vi "niWLAN - OPPO - 80211abgnGeneration(ref)_bc.vi"(0 "Rx Measurements Settings":T2 {"DSSS Data Rate (Mbps)" items=["1", "2", "5.5 CCK", "5.5 PBCC", "11 CCK", "11 PBCC", "22", "33"]; "OFDM Data Rate (Mbps)" items=["6", "9", "12", "18", "24", "36", "48", "54"]; "80211n PLCP Frame Format" items=["Mixed Format", "Greenfield Format"]; "Standard" items=["80211A/G/J/P OFDM", "80211B/G DSSS", "80211G DSSSOFDM", "80211N MIMOOFDM", "80211AC MIMOOFDM"]}, 5 "Without ACK ?":bool, 7 "Address String":string="00:90:4C:C5:12:38", 11 "error in":errorcluster) -> (4 "Cluster":T1, 15 "error out":errorcluster)   [LabVIEW 2012]
uses:
  TV/RW/Includes/WLAN - TV - RW - INC - Rx_PER_Wfm_Settings.ctl
  <vilib>/RF Toolkits/WLAN/generation/controls/wlanG version control.ctl
  <vilib>/RF Toolkits/WLAN/generation/niWLANG Create Multiple Channel Waveform (IQ Complex Cluster).vi
  <vilib>/RF Toolkits/WLAN/generation/niWLANG Create Single Channel Waveform (IQ Complex Cluster).vi
  <resource>/objmgr/niWLANGeneration.rc
panel:
  out "32bit integer":i32
  out "1/x":dbl
  in  "Boolean":bool
  in  "Idle Time (With Ack)":dbl
  in  "file path":path
  # "Hardware Configuration"
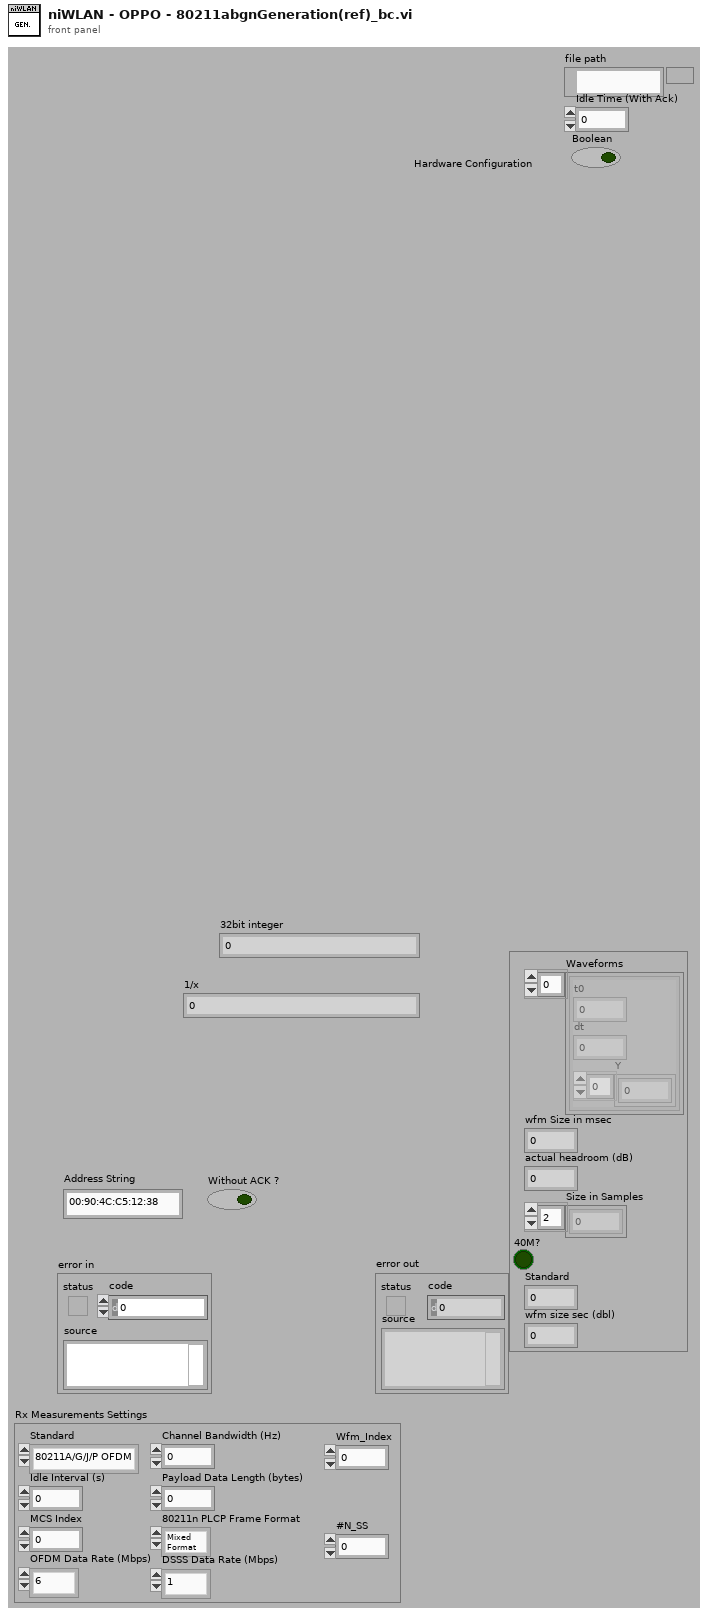
[diagram p1: front panel]
types:
  T1 = cluster{"Waveforms":cluster{"t0":dbl, "dt":dbl, "Y":cdb[]}[], "wfm Size in msec":i32, "actual headroom (dB)":dbl, "Size in Samples":i32[], "40M?":bool, "Standard ":i32, "wfm size sec (dbl)":dbl}
  T2 = typedef "WLAN - TV - RW - INC - Rx_PER_Wfm_Settings.ctl" = cluster{"Standard":i32, "Channel Bandwidth (Hz)":dbl, "Idle Interval (s)":dbl, "MCS Index":i32, "80211n PLCP Frame Format":i32, "Payload Data Length (bytes)":i32, "OFDM Data Rate (Mbps)":i32, "DSSS Data Rate (Mbps)":i32, "Wfm_Index":i32, "#N_SS":i32}
  T3 = typedef "wlanG version control.ctl" = i32
  T4 = typedef "wlanv1_generation refnum.ctl" = refnum<k20>
  T5 = typedef "wlanv1_Generation Refnum.ctl" = refnum<k20>
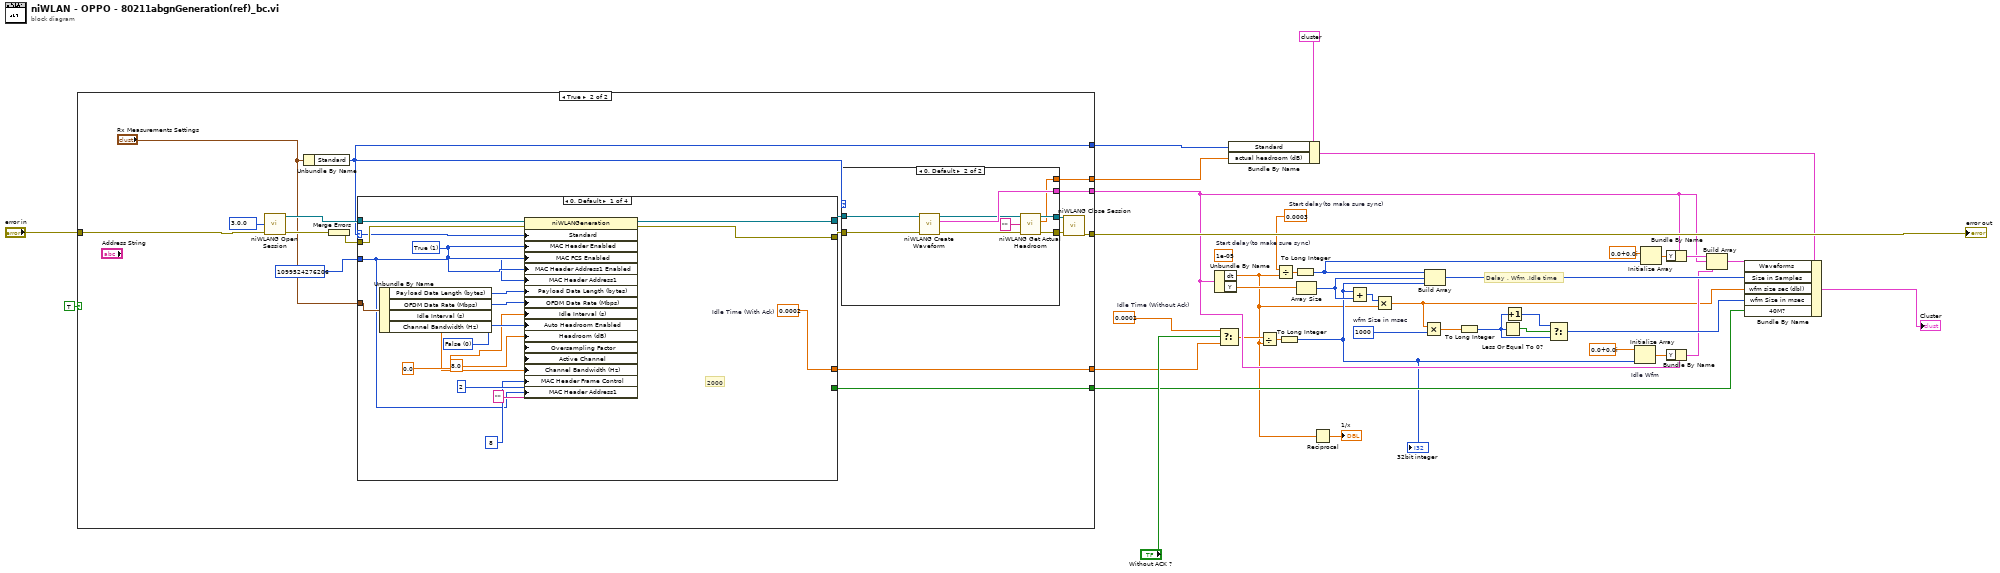
[diagram p0: block diagram]
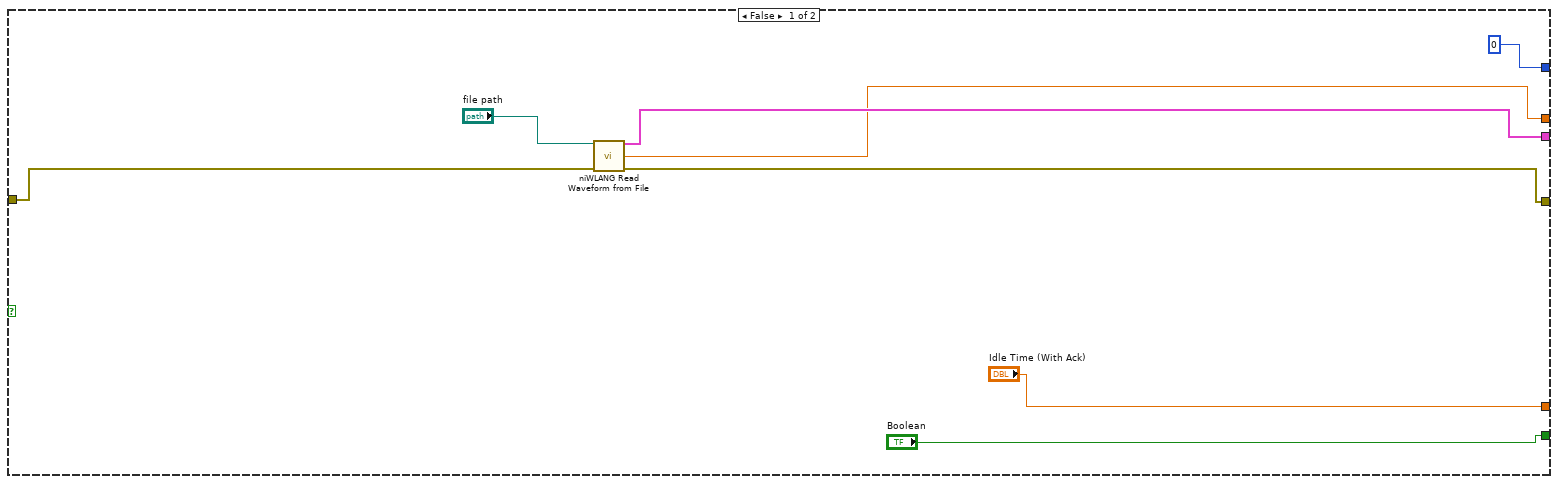
[diagram p2: hidden frame]
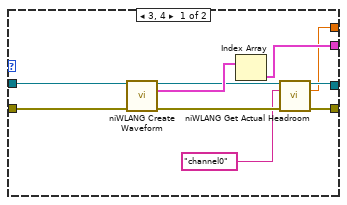
[diagram p3: hidden frame]
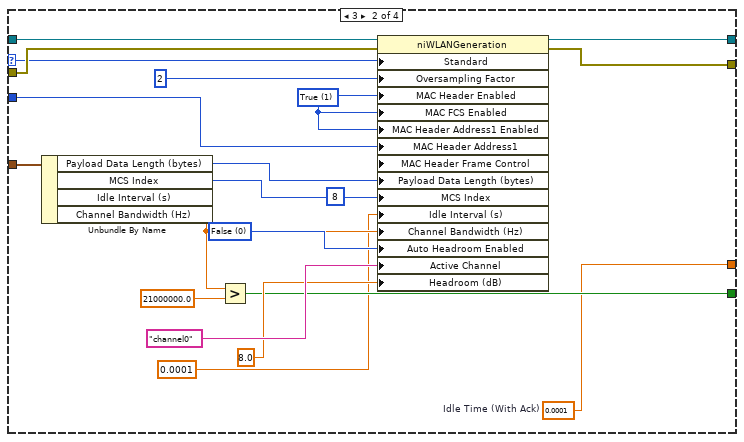
[diagram p4: hidden frame]
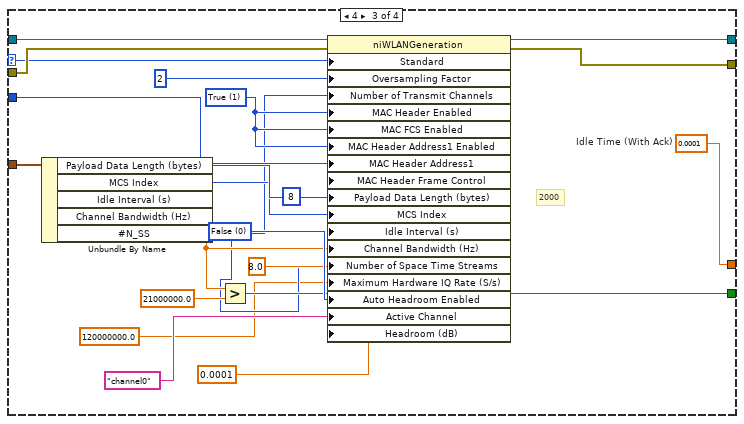
[diagram p5: hidden frame]
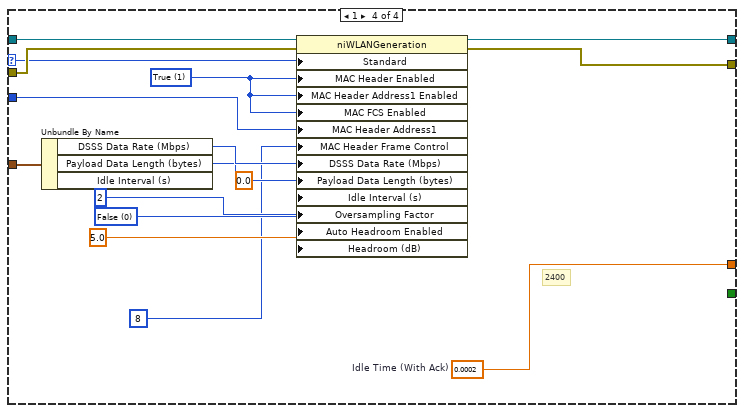
[diagram p6: hidden frame]
diagram:
  w5 = 0.0003  # Start delay(to make sure sync)
  (unwired) 1e-05  # Start delay(to make sure sync)
  w8 = 0.0002  # Idle Time (Without Ack)
  w17 = 1000  # wfm Size in msec
  # "Delay , Wfm ,Idle time"
  n1 = case shown="True" TRUE {
    tunnel: [w44 w64] -> w39
    tunnel: "error in" -> [w41 w63]
    tunnel: ["Boolean" w54] -> w25
    tunnel: [w46 w53] -> w18
    tunnel: [0 ("Standard") w52] -> w12
    tunnel: [w45 w51] -> w10
    tunnel: ["Idle Time (With Ack)" w50] -> w6
    frame False {
      n2 = call <vilib>:"niWLANG Read Waveform from File.vi"("file path"="file path", "error in"=w41) -> ("waveform"=w46:cluster{"t0":dbl, "dt":dbl, "Y":cdb[]}, "headroom (dB)"=w45:dbl, "error out"=w44:errorcluster)  [unwired: 9 in, 2 out]
    }
    frame True {
      w61 = T3 30000 items=["1.0.0"=10000, "2.0.0"=20000, "3.0.0"=30000] ("toolkit compatibility version")
      n3 = call <vilib>:"niWLANG Open Session.vi"("toolkit compatibility version"=w61, "error in"=w63) -> ("niwlan generation session"=w62:T4, "error out"=w60:errorcluster)  [unwired: 11 in, 1 out]
      n4 = Unbundle By Name("Rx Measurements Settings") -> ("Standard"=w52:i32)
      n5 = Merge Errors(w60) -> (w59:errorcluster)
      n6 = case shown="0, Default" w52 {
        selector: w52 -> [w96 w116 w138 w156]
        tunnel: w62 -> [w101 w120 w142 w159]
        tunnel: w59 -> [w100 w117 w139 w158]
        tunnel: [w99 w119 w141 w157] -> w56
        tunnel: [w98 w118 w140 w147] -> w55
        tunnel: u64 1099524276206 ("Address U64") -> [w84 w109 w131 w152]
        tunnel: "Rx Measurements Settings" -> [w90 w113 w135 w148]
        tunnel: [_ w105 w127 _] -> w54
        tunnel: [w88 w103 w125 w145] -> w50
        frame 0, Default {
          w88 = 0.0002  # Idle Time (With Ack)
          w94 = 0 items=["False", "True"] ("Auto Headroom Enabled")
          w97 = 1 items=["False", "True"] ("MAC Header Enabled")
          # "2000"
          n7 = Unbundle By Name(w90) -> ("Payload Data Length (bytes)"=w92:i32, "OFDM Data Rate (Mbps)"=w95:i32, "Channel Bandwidth (Hz)"=w86:dbl)  [unwired: 1 out]
          n8 = property class="niWLANGeneration"(reference=w101, error in=w100, "Standard"=w96, "MAC Header Enabled"=w97, "MAC FCS Enabled"=w97, "MAC Header Address1 Enabled"=w97, "MAC Header Address1"=w84, "Payload Data Length (bytes)"=w92, "OFDM Data Rate (Mbps)"=w95, "Idle Interval (s)"=0.0, "Auto Headroom Enabled"=w94, "Headroom (dB)"=8.0, "Oversampling Factor"=2, "Active Channel"="", "Channel Bandwidth (Hz)"=w86, "MAC Header Frame Control"=8, "MAC Header Address1"=w84) -> (reference out=w99:T4, error out=w98:errorcluster)
        }
        frame 3 {
          w103 = 0.0001  # Idle Time (With Ack)
          w112 = 0 items=["False", "True"] ("Auto Headroom Enabled")
          w121 = 1 items=["False", "True"] ("MAC Header Enabled")
          n9 = Unbundle By Name(w113) -> ("Payload Data Length (bytes)"=w115:i32, "MCS Index"=w114:i32, "Channel Bandwidth (Hz)"=w108:dbl)  [unwired: 1 out]
          n10 = Greater?(x=w108, y=21000000.0) -> (0:w105:bool)
          n11 = property class="niWLANGeneration"(reference=w120, error in=w117, "Standard"=w116, "Oversampling Factor"=2, "MAC Header Enabled"=w121, "MAC FCS Enabled"=w121, "MAC Header Address1 Enabled"=w121, "MAC Header Address1"=w109, "MAC Header Frame Control"=8, "Payload Data Length (bytes)"=w115, "MCS Index"=w114, "Idle Interval (s)"=0.0001, "Channel Bandwidth (Hz)"=w108, "Auto Headroom Enabled"=w112, "Active Channel"="channel0", "Headroom (dB)"=8.0) -> (reference out=w119:T4, error out=w118:errorcluster)
        }
        frame 4 {
          w125 = 0.0001  # Idle Time (With Ack)
          w134 = 0 items=["False", "True"] ("Auto Headroom Enabled")
          w143 = 1 items=["False", "True"] ("MAC Header Enabled")
          # "2000"
          n12 = Unbundle By Name(w135) -> ("Payload Data Length (bytes)"=w137:i32, "MCS Index"=w136:i32, "Channel Bandwidth (Hz)"=w130:dbl, "#N_SS"=w123:i32)  [unwired: 1 out]
          n13 = Greater?(x=w130, y=21000000.0) -> (0:w127:bool)
          n14 = property class="niWLANGeneration"(reference=w142, error in=w139, "Standard"=w138, "Oversampling Factor"=2, "Number of Transmit Channels"=w123, "MAC Header Enabled"=w143, "MAC FCS Enabled"=w143, "MAC Header Address1 Enabled"=w143, "MAC Header Address1"=w131, "MAC Header Frame Control"=8, "Payload Data Length (bytes)"=w137, "MCS Index"=w136, "Idle Interval (s)"=0.0001, "Channel Bandwidth (Hz)"=w130, "Number of Space Time Streams"=w123, "Maximum Hardware IQ Rate (S/s)"=120000000.0, "Auto Headroom Enabled"=w134, "Active Channel"="channel0", "Headroom (dB)"=8.0) -> (reference out=w141:T4, error out=w140:errorcluster)
        }
        frame 1 {
          w145 = 0.0002  # Idle Time (With Ack)
          w150 = 0 items=["False", "True"] ("Auto Headroom Enabled")
          w155 = 1 items=["False", "True"] ("OFDM Demod Enabled")
          # "2400"
          n15 = Unbundle By Name(w148) -> ("DSSS Data Rate (Mbps)"=w154:i32, "Payload Data Length (bytes)"=w153:i32)  [unwired: 1 out]
          n16 = property class="niWLANGeneration"(reference=w159, error in=w158, "Standard"=w156, "MAC Header Enabled"=w155, "MAC Header Address1 Enabled"=w155, "MAC FCS Enabled"=w155, "MAC Header Address1"=w152, "MAC Header Frame Control"=8, "DSSS Data Rate (Mbps)"=w154, "Payload Data Length (bytes)"=w153, "Idle Interval (s)"=0.0, "Oversampling Factor"=2, "Auto Headroom Enabled"=w150, "Headroom (dB)"=5.0) -> (reference out=w157:T4, error out=w147:errorcluster)
        }
      }
      n17 = case shown="0, Default" w52 {
        tunnel: [w69 w79] -> w57
        tunnel: w56 -> [w73 w83]
        tunnel: w55 -> [w74 w82]
        tunnel: [w67 w78] -> w58
        tunnel: [w71 w81] -> w53
        tunnel: [w65 w76] -> w51
        frame 3, 4 {
          n18 = call-poly <vilib>:"niWLANG Create Waveform.vi"("niwlan generation session"=w73, "error in"=w74) -> ("niwlan generation session out"=w70:T4, "output waveform"=w72:cluster{"t0":dbl, "dt":dbl, "Y":cdb[]}[], "error out"=w68:errorcluster)  [unwired: 10 in, 1 out]
          n19 = Index Array(array=w72) -> (element=w71:cluster{"t0":dbl, "dt":dbl, "Y":cdb[]})  [unwired: 1 in]
          n20 = call <vilib>:"niWLANG Get Actual Headroom.vi"("niwlan generation session"=w70, "active channel"="channel0", "error in"=w68) -> ("niwlan generation session out"=w69:T5, "actual headroom (dB)"=w65:dbl, "error out"=w67:errorcluster)  [unwired: 10 in]
        }
        frame 0, Default {
          n21 = call-poly <vilib>:"niWLANG Create Waveform.vi"("niwlan generation session"=w83, "error in"=w82) -> ("niwlan generation session out"=w80:T4, "output waveform"=w81:cluster{"t0":dbl, "dt":dbl, "Y":cdb[]}, "error out"=w77:errorcluster)  [unwired: 10 in, 1 out]
          n22 = call <vilib>:"niWLANG Get Actual Headroom.vi"("niwlan generation session"=w80, "active channel"="", "error in"=w77) -> ("niwlan generation session out"=w79:T5, "actual headroom (dB)"=w76:dbl, "error out"=w78:errorcluster)  [unwired: 10 in]
        }
      }
      n23 = call <vilib>:"niWLANG Close Session.vi"("niwlan generation session"=w57, "error in"=w58) -> ("error out"=w64:errorcluster)  [unwired: 13 in]
    }
  }
  "error out" <- w39
  n24 = Unbundle By Name(w18) -> ("dt"=w2:dbl, "Y"=w13:cdb[])
  n25 = Select(t=w8, s="Without ACK ?", f=w6) -> (s? t:f=w7:dbl)
  n26 = Bundle By Name(cluster=T1 {"Waveforms"=[{"t0"=0.0, "dt"=1.25e-08, "Y"=array[800 elements]}, {"t0"=0.0, "dt"=1.25e-08, "Y"=array[85448 elements]}], "wfm Size in msec"=1, "actual headroom (dB)"=0.0, "Size in Samples"=[10000000, 0], "40M?"=TRUE, "Standard "=3, "wfm size sec (dbl)"=0.0} ("Cluster"), "Standard"=w12, "actual headroom (dB)"=w10) -> (w11:T1)
  n27 = Divide(x=w7, y=w2) -> (x/y=w20:dbl)
  n28 = Divide(x=w5, y=w2) -> (x/y=w32:dbl)
  n29 = To Long Integer(number=w20) -> (32bit integer=w9:i32)
  "32bit integer" <- w9
  n30 = To Long Integer(number=w32) -> (32bit integer=w31:i32)
  n31 = Array Size(array=w13) -> (size(s)=w21:i32)
  n32 = Reciprocal(x=w2) -> (1/x=→"1/x":dbl)
  n33 = Add(x=w9, y=w21) -> (x+y=w19:i32)
  n34 = Multiply(x=w19, y=w2) -> (x*y=w15:dbl)
  n35 = Multiply(x=w15, y=w17) -> (x*y=w16:dbl)
  n36 = Build Array(w31, w21, w9) -> (w27:i32[])
  n37 = To Long Integer(number=w16) -> (32bit integer=w34:i32)
  n38 = Less Or Equal To 0?(x=w34) -> (x <= 0?=w35:bool)
  n39 = Increment(x=w34) -> (x+1=w33:i32)
  n40 = Select(t=w33, s=w35, f=w34) -> (s? t:f=w26:i32)
  n41 = Initialize Array "Idle Wfm"(cdb 0.0+0.0i ("element"), w9) -> (w23:cdb[])
  n42 = Initialize Array(cdb 0.0+0.0i ("element"), w31) -> (w30:cdb[])
  n43 = Bundle By Name(cluster=w18, "Y"=w30) -> (w29:cluster{"t0":dbl, "dt":dbl, "Y":cdb[]})
  n44 = Bundle By Name(cluster=w18, "Y"=w23) -> (w22:cluster{"t0":dbl, "dt":dbl, "Y":cdb[]})
  n45 = Build Array(w29, w18, w22) -> (w28:cluster{"t0":dbl, "dt":dbl, "Y":cdb[]}[])
  n46 = Bundle By Name(cluster=w11, "Waveforms"=w28, "Size in Samples"=w27, "wfm size sec (dbl)"=w15, "wfm Size in msec"=w26, "40M?"=w25) -> (→"Cluster":T1)
